vi "Write Data to Conn.vi"(8 "error in (no error)":errorcluster, 9 "Data":string, 10 "MetaData":string, 11 "TCP Connection in":refnum<class "TCP Connection.lvclass">) -> (0 "error out":errorcluster, 3 "TCP Connection out":refnum<class "TCP Connection.lvclass">)   [LabVIEW 2012, in "TCP Classes.lvlib" / "TCP Connection.lvclass"]
uses:
  TCP Connection.lvclass
  TCP Connection.lvclass/TCP Connection.ctl
  <userlib>/STM/TCP/stm_TCP Write Options.ctl
  <userlib>/STM/TCP/STM Write Message (TCP).vi
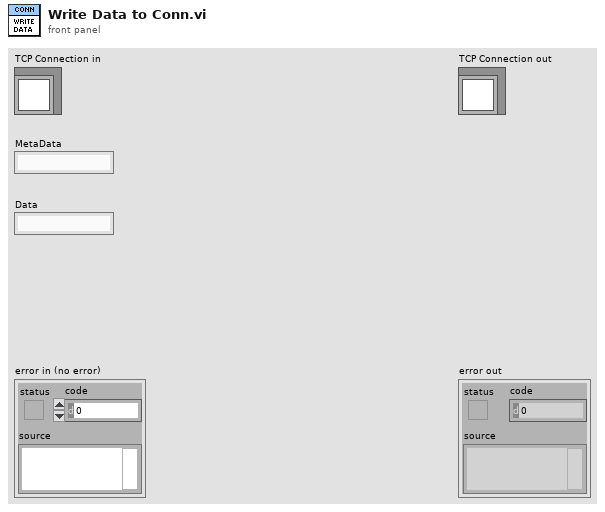
[diagram p1: front panel]
types:
  T1 = typedef "stm_TCP Write Options.ctl" = cluster{"Ignore Timeout Error":bool, "timeout ms (1000)":i32}
  T2 = typedef "stm_TCP Connection Info.ctl" = cluster{"connection ID":refnum<k5>, "Meta data":T3[]}
  T3 = typedef "stm_MetaDataElement.ctl" = string
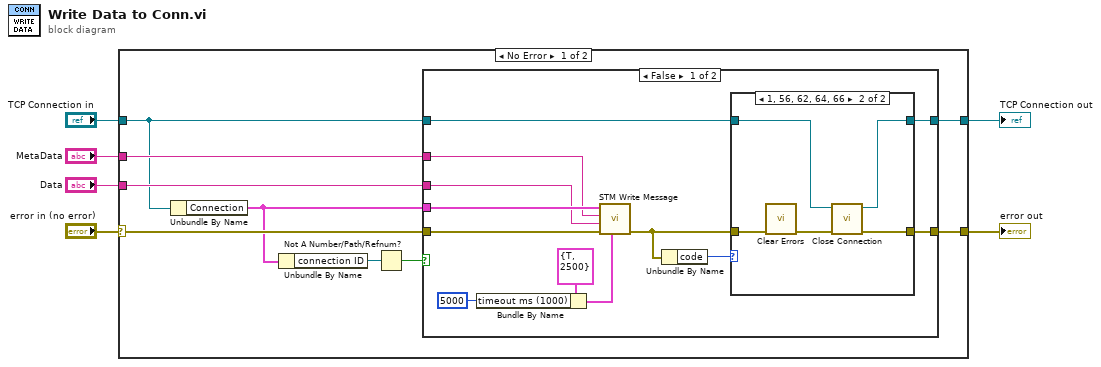
[diagram p0: block diagram]
diagram:
  n1 = case shown="No Error" "error in (no error)" {
    selector: "error in (no error)" -> [w9 w38]
    tunnel: [w14 w38] -> w5
    tunnel: [w13 w37] -> w3
    tunnel: "TCP Connection in" -> [w10 w37]
    tunnel: "MetaData" -> [w12 _]
    tunnel: "Data" -> [w11 _]
    frame No Error {
      n2 = Unbundle By Name(w10) -> ("Connection"=w8:T2)
      n3 = Unbundle By Name(w8) -> ("connection ID"=w7:refnum<k5>)
      n4 = Not A Number/Path/Refnum?(number/path/refnum=w7) -> (NaN/Path/Refnum?=w15:bool)
      n5 = case shown="False" w15 {
        tunnel: [w22 w35] -> w14
        tunnel: w9 -> [w27 w35]
        tunnel: w8 -> [w26 _]
        tunnel: w10 -> [w21 w36]
        tunnel: [w20 w36] -> w13
        tunnel: w12 -> [w17 _]
        tunnel: w11 -> [w16 _]
        frame False {
          n6 = Bundle By Name(cluster=T1 {"Ignore Timeout Error"=TRUE, "timeout ms (1000)"=2500} ("Options"), "timeout ms (1000)"=5000) -> (w23:T1)
          n7 = call-poly <userlib>:"STM Write Message.vi"("Options"=w23, "error in (no error)"=w27, "Data"=w16, "Name"=w17, "Connection Info"=w26) -> ("error out"=w19:errorcluster)  [unwired: 5 in, 1 out]
          n8 = Unbundle By Name(w19) -> ("code"=w18:i32)
          n9 = case shown="1, 56, 62, 64, 66" w18 {
            tunnel: w19 -> [w28 w34]
            tunnel: [w28 w32] -> w22
            tunnel: w21 -> [w29 w31]
            tunnel: [w29 w30] -> w20
            frame Default {
            }
            frame 1, 56, 62, 64, 66 {
              n10 = call <vilib>:"Clear Errors.vi"("error in (no error)"=w34) -> ("error out"=w33:errorcluster)  [unwired: 6 in]
              n11 = call "Close Connection.vi"("error in (no error)"=w33, "TCP Connection in"=w31) -> ("error out"=w32:errorcluster, "TCP Connection out"=w30:refnum<class "TCP Connection.lvclass">)  [unwired: 8 in]
            }
          }
        }
        frame True {
        }
      }
    }
    frame Error {
    }
  }
  "error out" <- w5
  "TCP Connection out" <- w3
